vi "sub_FEA_Model_for_LEMP.vi"(1 "Setup Parameters":T1) -> (0 "LEMP":T2)   [LabVIEW 2021]
panel:
  out "size(s)":i32[](array[numeric])
  # "Input"
  # "Output"
  # "This VI acquires the required input cluster for the Sub_online_LEMP_Update.vi, this VI calls on SciPy.linalg.eigh() due to issues with the standard \"General Eigenvalues and Eigenvectors.vi\" outputting inappropriately scaled eigenvectors for the LEMP. Additionally the Bitedness of this installation of LabVIEW does not match with Python so direct python calls were similarly unavailable. The workaround involved a saving the matrices in a text format command line calling the SciPy eigh function saving that output as a text file, then load the output file in to memory (See Sub_Python_cmd_eigh.vi, getEigenCommandPrompt.py , mass.lvm, stiff.lvm,eigenvalues.txt, eigenvectors.txt).\n\n              - Alexander Vereen AFRL Summer scholars 2022"
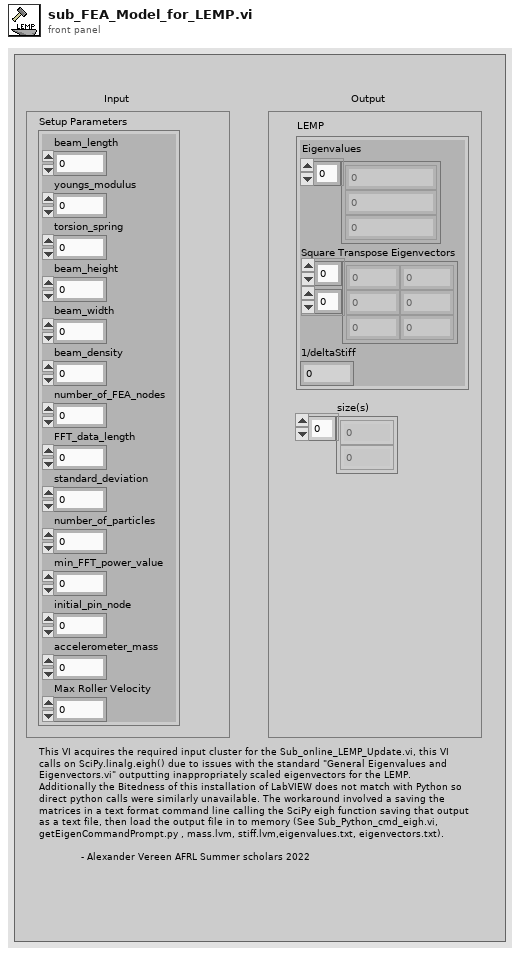
[diagram p1: front panel]
types:
  T1 = cluster{"beam_length":dbl, "youngs_modulus":dbl, "torsion_spring":dbl, "beam_height":dbl, "beam_width":dbl, "beam_density":dbl, "number_of_FEA_nodes":i32, "FFT_data_length":i32, "standard_deviation":dbl, "number_of_particles":i32, "min_FFT_power_value":dbl, "initial_pin_node":i32, "accelerometer_mass":dbl, "Max Roller Velocity":dbl}
  T2 = cluster{"Eigenvalues":dbl[], "Square Transpose Eigenvectors":dbl[][], "1/deltaStiff":dbl}
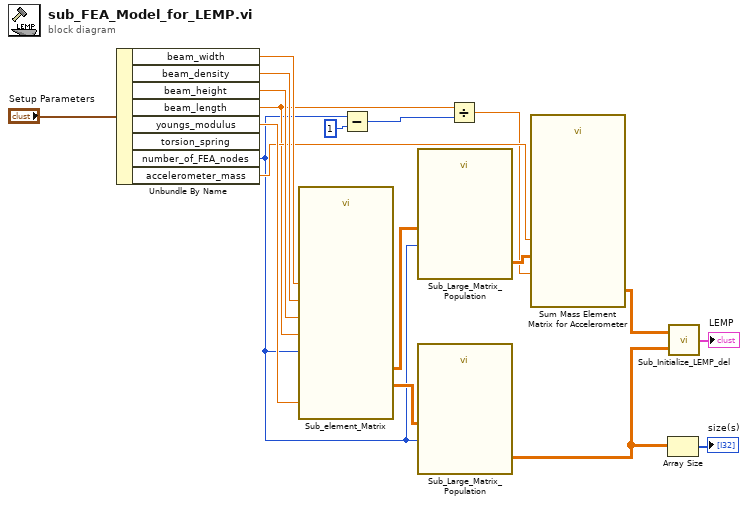
[diagram p0: block diagram]
diagram:
  n1 = Unbundle By Name("Setup Parameters") -> ("beam_width"=w13:dbl, "beam_density"=w14:dbl, "beam_height"=w15:dbl, "beam_length"=w8:dbl, "youngs_modulus"=w16:dbl, "number_of_FEA_nodes"=w6:i32, "accelerometer_mass"=w9:dbl)  [unwired: 1 out]
  n2 = call "Sub_element_Matrix.vi"("Length of Beam"=w8, "Young's Modulus"=w16, "No. of Nodes"=w6, "Height"=w15, "Width"=w13, "Density"=w14) -> ("M Element Matrix"=w17:dbl[][], "K Element Matrix"=w18:dbl[][])  [unwired: 11 in, 1 out]
  n3 = Subtract(x=w6, y=1) -> (x-y=w11:i32)
  n4 = call "Sub_Large_Matrix_Population.vi"("No. of Nodes"=w6, "Element Matrix"=w17) -> ("Matrix w/o BC"=w12:dbl[][])  [unwired: 9 in]
  n5 = call "Sub_Large_Matrix_Population.vi"("No. of Nodes"=w6, "Element Matrix"=w18) -> ("Matrix w/o BC"=w2:dbl[][])  [unwired: 9 in]
  n6 = Divide(x=w8, y=w11) -> (x/y=w7:dbl)
  n7 = call "Sum Mass Element Matrix for Accelerometer.vi"("Matrix w/o BC"=w12, "accelerometer_mass"=w9, "Element Length"=w7) -> ("Matrix W/ Accelerometer"=w5:dbl[][])  [unwired: 8 in]
  n8 = Array Size(array=w2) -> (size(s)=→"size(s)":i32[])
  n9 = call "Sub_Initialize_LEMP_del.vi"("Stiff"=w2, "Mass"=w5) -> ("LEMP"=→"LEMP":T2)
